vi "stringmatch.vi"() -> ()   [LabVIEW 2019]
panel:
  out "Numeric":dbl
  out "match substring":string
  in  "String":string
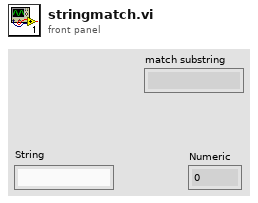
[diagram p1: front panel]
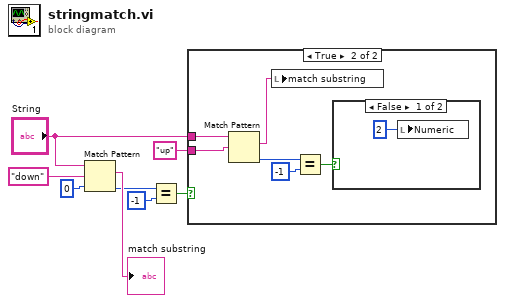
[diagram p0: block diagram]
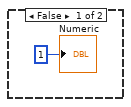
[diagram p2: hidden frame]
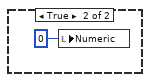
[diagram p3: hidden frame]
diagram:
  n1 = Match Pattern(string="String", regular expression="down", offset (0)=0) -> (match substring=→"match substring":string, offset past match=w5:i32)  [unwired: 2 out]
  n2 = Equal?(x=w5, y=-1) -> (x = y?=w3:bool)
  n3 = case shown="True" w3 {
    tunnel: "String" -> [_ w15]
    tunnel: "up" ("regular expression") -> [_ w14]
    frame False {
      "Numeric" <- 1
    }
    frame True {
      n4 = Match Pattern(string=w15, regular expression=w14) -> (match substring=w10:string, offset past match=w13:i32)  [unwired: 1 in, 2 out]
      n5 = local write "match substring"(w10) -> ()
      n6 = Equal?(x=w13, y=-1) -> (x = y?=w11:bool)
      n7 = case shown="False" w11 {
        frame False {
          n8 = local write "Numeric"(2) -> ()
        }
        frame True {
          n9 = local write "Numeric"(0) -> ()
        }
      }
    }
  }
